vi "stop_movie.vi"(8 "error in (no error)":errorcluster, 11 "DataCollectionDL091104Scaffold in":refnum<class "DataCollectionDL091104Scaffold.lvclass">) -> (0 "error out":errorcluster, 3 "DataCollectionDL091104Scaffold out":refnum<class "DataCollectionDL091104Scaffold.lvclass">)   [LabVIEW 2010, in "DataCollectionDL091104Scaffold.lvclass"]
uses:
  DataCollectionDL091104Scaffold.lvclass
  DataCollectionDL091104Scaffold.lvclass/DataCollectionDL091104Scaffold.ctl
  common/classes/ErrorController/ErrorController/class_data.vi
  common/classes/ErrorController/ErrorController/ErrorController.lvclass
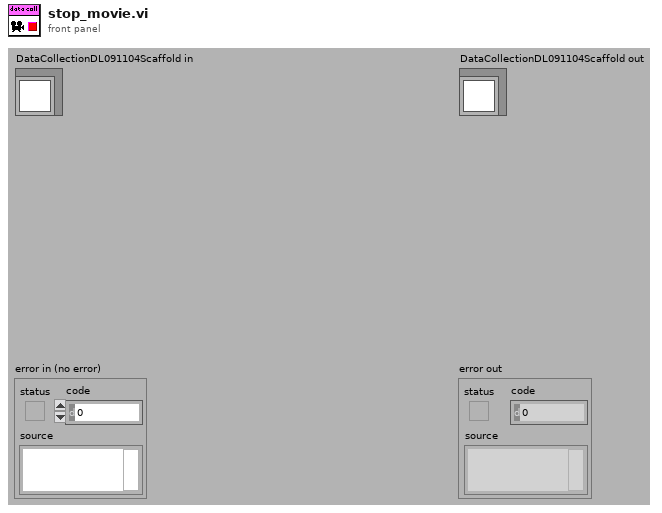
[diagram p1: front panel]
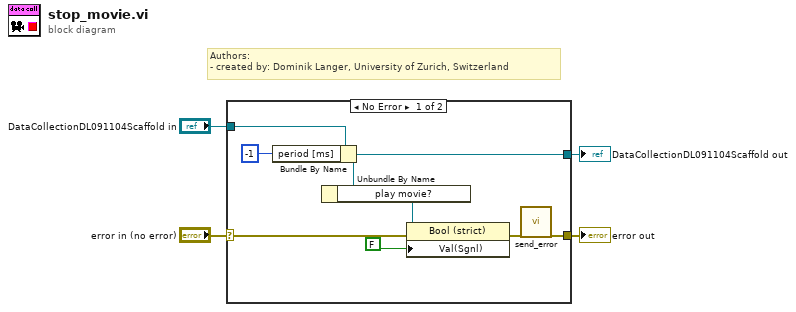
[diagram p0: block diagram]
diagram:
  # "Authors: \n- created by: Dominik Langer, University of Zurich, Switzerland"
  n1 = case shown="No Error" "error in (no error)" {
    selector: "error in (no error)" -> [w7 w14]
    tunnel: [w5 w14] -> w3
    tunnel: [w10 w13] -> w1
    tunnel: "DataCollectionDL091104Scaffold in" -> [w12 w13]
    frame No Error {
      n2 = Bundle By Name(cluster=w12, "period [ms]"=-1) -> (w10:refnum<class "DataCollectionDL091104Scaffold.lvclass">)
      n3 = Unbundle By Name(w10) -> ("play movie?"=w9:refnum<vi>)
      n4 = property class="Bool (strict)"(reference=w9, error in=w7, "Val(Sgnl)"=FALSE) -> (error out=w6:errorcluster)  [unwired: 1 out]
      n5 = call "send_error.vi"("error in (no error)"=w6) -> ("error out"=w5:errorcluster)  [unwired: 10 in]
    }
    frame Error {
    }
  }
  "error out" <- w3
  "DataCollectionDL091104Scaffold out" <- w1
